vi "GVMWHorst_ECD.vi"() -> ()   [LabVIEW 2017]
panel:
  in  "MWHorst":dbl[](array[numeric])
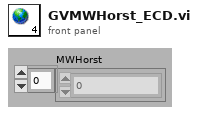
[diagram p1: front panel]
diagram:
